vi "Add Item to Tree with custom Symbol LV2012 NIVerified.vi"() -> ()   [LabVIEW 2012]
doc: "Demonstrates how to add an image as a symbol to a tree control"
panel:
  in  "Get Symbol Picture":bool
  out "Symbol Picture":picture
  in  "stop":bool
  in  "Tree":string(tree)="PIC"
  in  "Add":bool
  in  "Child Text":string[](array[string])=["text1", "text2"]
  in  "Left Cell String":string="CVI"
  in  "Symbol Image":u16(ring) items=["CVI"=41, "DIAdem"=42, "FPGA"=43, "LabVIEW"=44, "RealTime"=45, "SignalExpress"=46, "VeriStand"=47]
  # "Overview: Demonstrates how to add an image as a symbol to a tree control\nRequirements: LabVIEW 2012 Base Development System (or compatible)\nInstructions: \n1. Run the VI\n2. Select the desired Symbol Image\n3. Click 'Add' to add the symbol with the Left Cell String and the Child Text to the Tree control\n4. Click 'Get Symbol Picture' to display the Symbol Picture in full resolution"
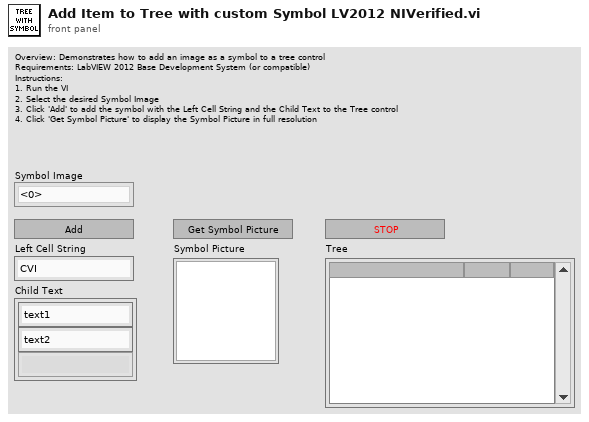
[diagram p1: front panel]
types:
  T1 = typedef "imagedata.ctl" = cluster{"image type":i32, "image depth":i32, "image":u8[], "mask":u8[], "colors":u32[], "Rectangle":cluster{"left":i16, "top":i16, "right":i16, "bottom":i16}}
  T2 = cluster{"filename without extension":string, i32}
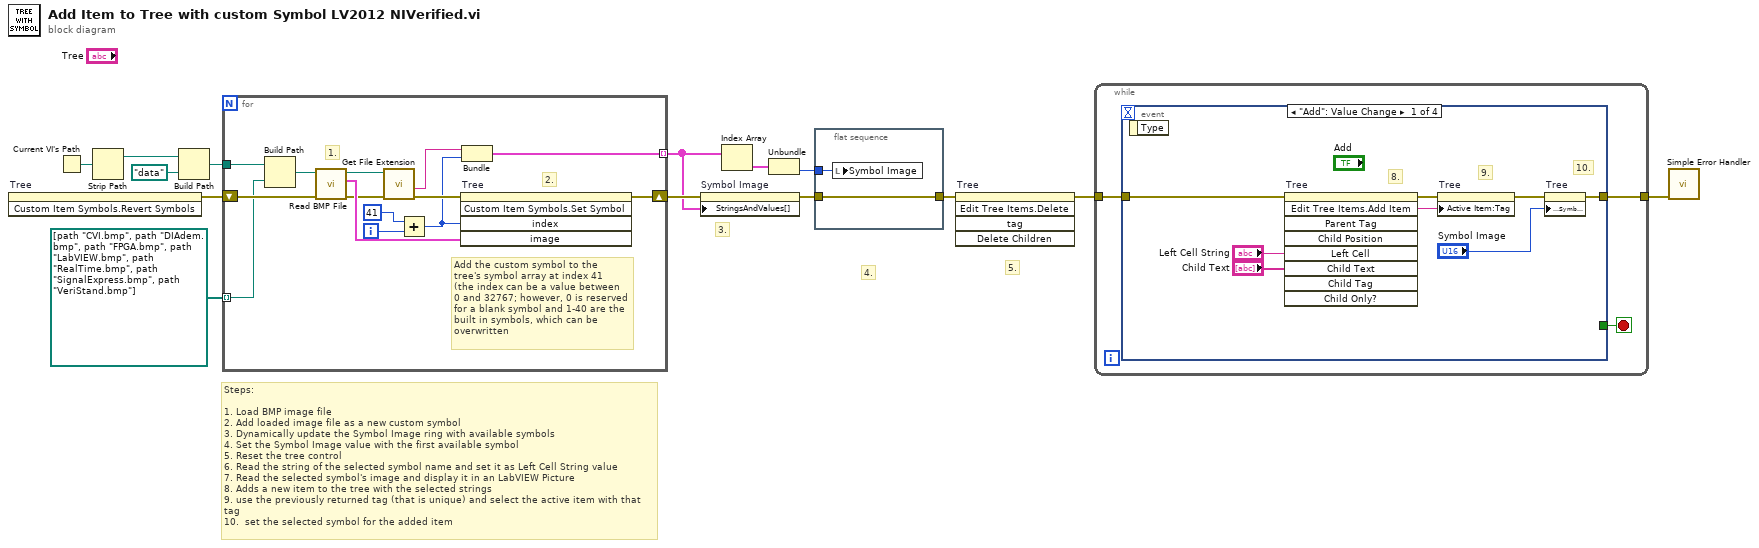
[diagram p0: block diagram]
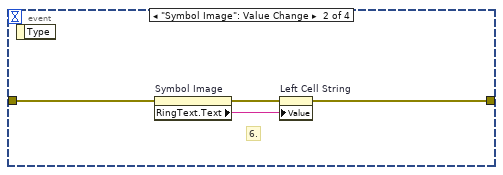
[diagram p2: hidden frame]
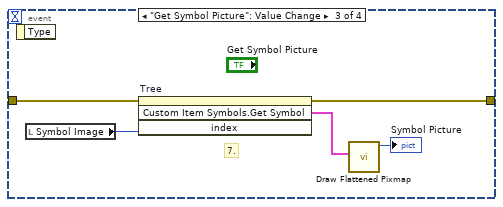
[diagram p3: hidden frame]
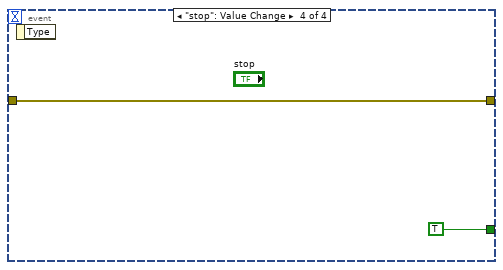
[diagram p4: hidden frame]
diagram:
  # "5."
  # "4."
  # "3."
  # "Steps:\n\n1. Load BMP image file\n2. Add loaded image file as a new custom symbol\n3. Dynamically update the Symbol Image ring with available symbols\n4. Set the Symbol Image value with the first available symbol\n5. Reset the tree control\n6. Read the string of the selected symbol name and set it as Left Cell String value\n7. Read the selected symbol's image and display it in an LabVIEW Picture\n8. Adds a new item to the tree with the selected strings\n9. use the previously returned tag (that is unique) and select the active item with that tag\n10.  set the selected symbol for the added item"
  n1 = invoke on="Tree" class="TreeControl (strict)" method="Custom Item Symbols.Revert Symbols"() -> (error out=w9:errorcluster)  [unwired: 3 in, 2 out]
  n2 = Current VI's Path() -> (path=w13:path)
  n3 = Strip Path(path=w13) -> (stripped path=w12:path)  [unwired: 1 out]
  n4 = Build Path(base path=w12, name or relative path=path "data" ("stripped path")) -> (appended path=w10:path)
  n5 = for {
    tunnel: w10 -> [w23]
    shift-right: [w28] -> w7
    shift-left: w9 -> [w26]
    tunnel: path[] [path "CVI.bmp", path "DIAdem.bmp", path "FPGA.bmp", path "LabVIEW.bmp", path "RealTime.bmp", path "SignalExpress.bmp", path "VeriStand.bmp"] -> [w21] mode=indexing
    tunnel: [w15] -> w5 mode=indexing
    i -> [w24]
    # "2."
    # "1."
    # "Add the custom symbol to the \ntree's symbol array at index 41 \n(the index can be a value between \n0 and 32767; however, 0 is reserved\nfor a blank symbol and 1-40 are the\nbuilt in symbols, which can be\noverwritten"
    n6 = Build Path(base path=w23, name or relative path=w21) -> (appended path=w22:path)
    n7 = call <vilib>:"Read BMP File.vi"("error in (no error)"=w26, "path to BMP file"=w22) -> ("error out"=w19:errorcluster, "image data"=w27:T1, "path"=w20:path)  [unwired: 7 in]
    n8 = call <vilib>:"Get File Extension.vi"("error in (no error)"=w19, "file"=w20) -> ("error out"=w18:errorcluster, "filename without extension"=w16:string)  [unwired: 6 in, 2 out]
    n9 = Add(x=41 ("Index"), y=w24) -> (x+y=w17:i32)
    n10 = invoke on="Tree" class="TreeControl (strict)" method="Custom Item Symbols.Set Symbol"(error in=w18, "index"=w17, "image"=w27) -> (error out=w28:errorcluster)  [unwired: 2 in, 4 out]
    n11 = Bundle("filename without extension"=w16, w17) -> (w15:T2)  [unwired: 1 in]
  }
  n12 = property on="Symbol Image" class="Ring (strict)"(error in=w7, "StringsAndValues[]"=w5) -> (error out=w1:errorcluster)  [unwired: 1 in, 1 out]
  n13 = Index Array(array=w5) -> (element=w4:T2)  [unwired: 1 in]
  n14 = Unbundle(w4) -> (w3:i32)  [unwired: 1 out]
  n15 = flat-sequence {
    tunnel: w3 -> [w30]
    tunnel: [w29] -> w2
    tunnel: w1 -> [w29]
    frame #0 {
      n16 = local write "Symbol Image"(w30) -> ()
    }
  }
  n17 = invoke on="Tree" class="TreeControl (strict)" method="Edit Tree Items.Delete"(error in=w2) -> (error out=w6:errorcluster)  [unwired: 4 in, 4 out]
  n18 = while {
    tunnel: [w33] -> w14
    tunnel: w6 -> [w32]
    stop <- w31 stop-if-true
    n19 = event shown="[0] \"Add\": Value Change" {
      selector: _ -> [_ _ _ _]
      dyn-events: _ -> [_ _ _ _]
      timeout: _ -> [_ _ _ _]
      tunnel: [w37 w42 w47 w51] -> w33
      tunnel: w32 -> [w34 w45 w48 w51]
      tunnel: [_ _ _ TRUE] -> w31
      event "Add": Value Change {
        # "10."
        # "9."
        # "8."
        n20 = event-data() -> ()  [unwired: 1 in, 1 out]
        n21 = invoke on="Tree" class="TreeControl (strict)" method="Edit Tree Items.Add Item"(error in=w34, "Left Cell"="Left Cell String", "Child Text"="Child Text") -> (error out=w40:errorcluster, "Edit Tree Items:Add Item"=w38:string)  [unwired: 6 in, 7 out]
        n22 = property on="Tree" class="Tree (strict)"(error in=w40, "Active Item:Tag"=w38) -> (error out=w39:errorcluster)  [unwired: 1 in, 1 out]
        n23 = property on="Tree" class="Tree (strict)"(error in=w39, "Active Item:Symbol Index"="Symbol Image") -> (error out=w37:errorcluster)  [unwired: 1 in, 1 out]
      }
      event "Symbol Image": Value Change {
        # "6."
        n24 = event-data() -> ()  [unwired: 1 in, 1 out]
        n25 = property on="Symbol Image" class="Ring (strict)"(error in=w45) -> (error out=w44:errorcluster, "RingText.Text"=w43:string)  [unwired: 1 in, 1 out]
        n26 = property on="Left Cell String" class="Str"(error in=w44, "Value"=w43) -> (error out=w42:errorcluster)  [unwired: 1 in, 1 out]
      }
      event "Get Symbol Picture": Value Change {
        # "7."
        n27 = event-data() -> ()  [unwired: 1 in, 1 out]
        n28 = local read "Symbol Image"() -> (w46:u16)
        n29 = invoke on="Tree" class="TreeControl (strict)" method="Custom Item Symbols.Get Symbol"(error in=w48, "index"=w46) -> (error out=w47:errorcluster, "Custom Glyphs:Get Glyph"=w50:T1)  [unwired: 2 in, 2 out]
        n30 = call <vilib>:"Draw Flattened Pixmap.vi"("image data"=w50) -> ("new picture"=→"Symbol Picture":picture)  [unwired: 8 in]
      }
      event "stop": Value Change {
        n31 = event-data() -> ()  [unwired: 1 in, 1 out]
      }
    }
  }
  n32 = call <vilib>:"Simple Error Handler.vi"("error in (no error)"=w14) -> ()  [unwired: 4 in, 5 out]
